vi "New Object on Parent Wire.vi"(8 "error in":errorcluster) -> (0 "error out":errorcluster, 3 "Node.lvclass":refnum<class "Node.lvclass">)   [LabVIEW 2014, in "Text Node.lvclass"]
uses:
  Text Node.lvclass
  Node_class/Node.lvclass
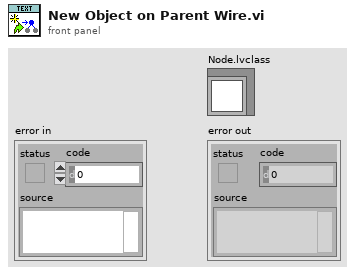
[diagram p1: front panel]
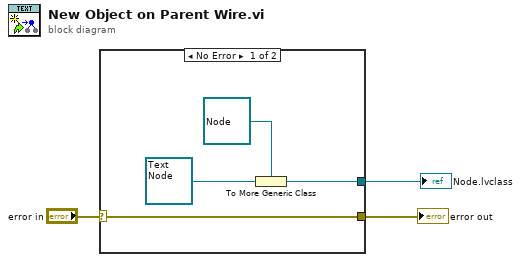
[diagram p0: block diagram]
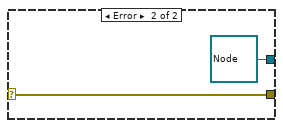
[diagram p2: hidden frame]
diagram:
  n1 = case shown="No Error" "error in" {
    selector: "error in" -> [w7 w9]
    tunnel: [w7 w9] -> w2
    tunnel: [w5 refnum<class "Node.lvclass"> refnum ("Node.lvclass")] -> w1
    frame No Error {
      n2 = To More Generic Class(target class=refnum<class "Node.lvclass"> refnum ("Node.lvclass"), reference=refnum<class "Text Node.lvclass"> refnum ("Text Node.lvclass")) -> (generic class reference=w5:refnum<class "Node.lvclass">)
    }
    frame Error {
    }
  }
  "error out" <- w2
  "Node.lvclass" <- w1
